vi "Auto Check for Ball.vi"(11 "Run?":bool) -> (3 "Done":bool)   [LabVIEW 2013]
panel:
  out "Averaged Value":dbl
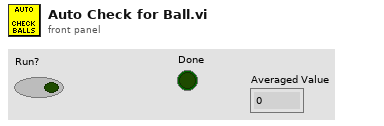
[diagram p1: front panel]
types:
  T1 = typedef "WPI_AnalogChannelDevRef.ctl" = cluster{"DevStatus":errorcluster, "Analog Module":T2, "Analog Channel":T3}
  T2 = typedef "FPGA_TypedefAnalogModule.ctl" = enum16{"Analog Module 1", "Analog Module 2"}
  T3 = typedef "FPGA_AIChannel.ctl" = enum8{"AI 1", "AI 2", "AI 3", "AI 4", "AI 5", "AI 6", "AI 7", "AI 8", "Invalid"}
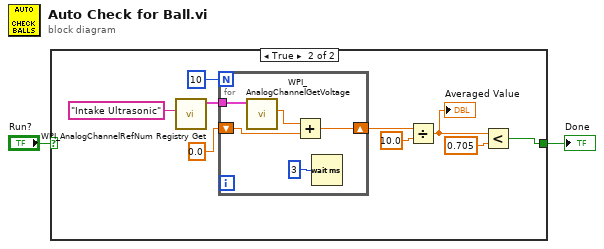
[diagram p0: block diagram]
diagram:
  n1 = case shown="True" "Run?" {
    selector: "Run?" -> [w3 _]
    tunnel: [w3 w10] -> w1
    frame False {
    }
    frame True {
      n2 = call <vilib>:"WPI_AnalogChannelRefNum Registry Get.vi"("refnum name"="Intake Ultrasonic") -> ("AIDeviceRef"=w8:T1)  [unwired: 9 in, 1 out]
      n3 = for {
        N: 10 -> [_]
        tunnel: w8 -> [w17]
        shift-right: [w14] -> w6
        shift-left: 0.0 ("Voltage") -> [w16]
        n4 = call <vilib>:"WPI_AnalogChannelGetVoltage.vi"("AIDeviceRef"=w17) -> ("Voltage"=w15:dbl)  [unwired: 8 in, 2 out]
        n5 = Add(x=w15, y=w16) -> (x+y=w14:dbl)
        n6 = Wait (ms)(milliseconds to wait=u32 3) -> ()  [unwired: 1 out]
      }
      n7 = Divide(x=w6, y=10.0) -> (x/y=w4:dbl)
      "Averaged Value" <- w4
      n8 = Less?(x=w4, y=0.705) -> (x < y?=w10:bool)
    }
  }
  "Done" <- w1
